vi "Motic Get Frame Format.vi"(8 "error in (no error)":errorcluster, 11 "camera":i32) -> (0 "error out":errorcluster, 1 "components per pixel":i32, 2 "frame format":u32(ring) items=["GRBG", "BGGR", "GBRG", "RGGB", "RGB", "BGR", "Monochrome"], 3 "camera out":i32)   [LabVIEW 2012, in "MoticApi.lvlib"]
doc: "MOTICAPI MUCam_Format Motic_GetFrameFormat(MUCam_Handle camera);"
uses:
  MoticApi.lvlib
  MoticApi.dll
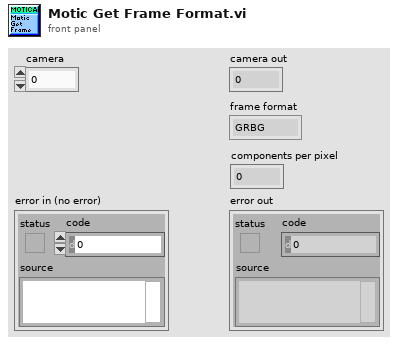
[diagram p1: front panel]
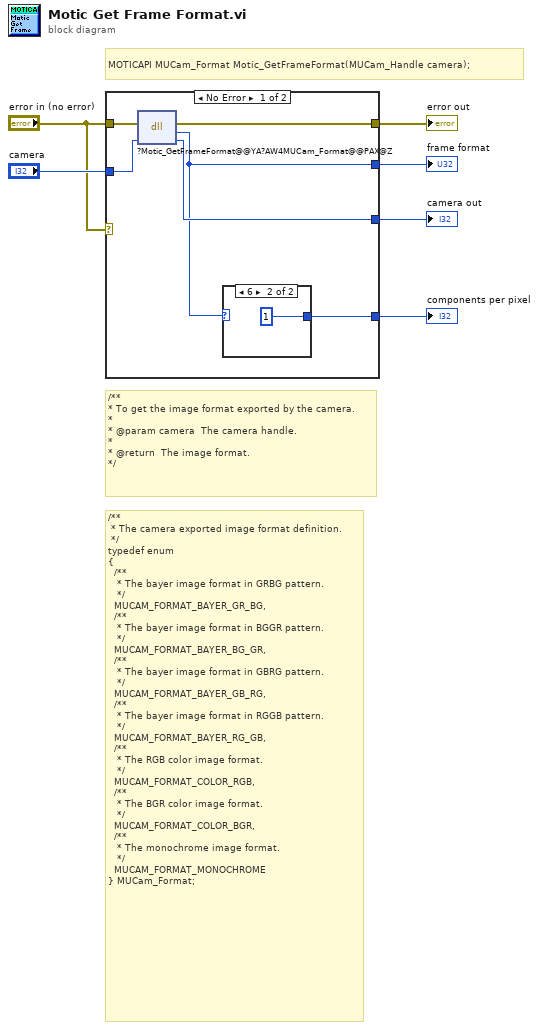
[diagram p0: block diagram]
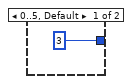
[diagram p2: hidden frame]
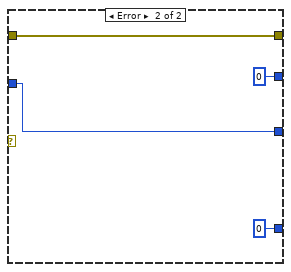
[diagram p3: hidden frame]
diagram:
  # "/**\n * The camera exported image format definition.\n */\ntypedef enum\n{\n  /**\n   * The bayer image format in GRBG pattern.\n   */\n  MUCAM_FORMAT_BAYER_GR_BG,\n  /**\n   * The bayer image format in BGGR pattern.\n   */\n  MUCAM_FORMAT_BAYER_BG_GR,\n  /**\n   * The bayer image format in GBRG pattern.\n   */\n  MUCAM_FORMAT_BAYER_GB_RG,\n  /**\n   * The bayer image format in RGGB pattern.\n   */\n  MUCAM_FORMAT_BAYER_RG_GB,\n  /**\n   * The RGB color image format.\n   */\n  MUCAM_FORMAT_COLOR_RGB,\n  /**\n   * The BGR color image format.\n   */\n  MUCAM_FORMAT_COLOR_BGR,\n  /**\n   * The monochrome image format.\n   */\n  MUCAM_FORMAT_MONOCHROME\n} MUCam_Format;"
  # "/**\n* To get the image format exported by the camera.\n*\n* @param camera  The camera handle.\n*\n* @return  The image format.\n*/"
  # "MOTICAPI MUCam_Format Motic_GetFrameFormat(MUCam_Handle camera);"
  n1 = case shown="No Error" "error in (no error)" {
    tunnel: "camera" -> [w12 w17]
    tunnel: [w11 w17] -> w5
    tunnel: "error in (no error)" -> [w10 w18]
    tunnel: [w9 w18] -> w4
    tunnel: [w8 0] -> w3
    tunnel: [w7 u32 0 ("return type")] -> w2
    frame No Error {
      n2 = dll-call lib="C:/Users/TTS-Digital/Desktop/MoticApi/MoticApi_git/MoticApi/MoticApi.*" fn="?Motic_GetFrameFormat@@YA?AW4MUCam_Format@@PAX@Z"(error in=w10, "camera"=w12) -> (error out=w9:errorcluster, "return type"=w7:u32, "camera"=w11:i32)  [unwired: 2 in, 1 out]
      n3 = case shown="6" w7 {
        tunnel: [3 1] -> w8
        frame 0..5, Default {
        }
        frame 6 {
        }
      }
    }
    frame Error {
    }
  }
  "camera out" <- w5
  "error out" <- w4
  "components per pixel" <- w3
  "frame format" <- w2
